vi "Initialize.vi"(8 "error in (no error)":errorcluster, 9 "Reset (True)":bool=TRUE, 10 "ID Query (True)":bool=TRUE, 11 "VISA resource name":refnum<visa-resource-name>) -> (0 "error out":errorcluster, 3 "VISA resource name out":refnum<visa-resource-name>)   [LabVIEW 2020, in "Library Instrument & Equipement.lvlib" / "Library Multimeter.lvlib" / "RIGOL DM3058.lvlib"]
doc: "Establishes communication with the instrument and optionally performs an instrument identification query and/or an instrument reset. It also places the instrument in a default state needed for other instrument driver operations. Therefore, call this VI before calling other instrument driver VIs for this instrument. Generally, you need to call the Initialize VI only once at the beginning of an application."
uses:
  RIGOL DM3058.lvlib
panel:
  # "(c) 2009-2015, RIGOL Technologies, Inc.  All Rights Reserved."
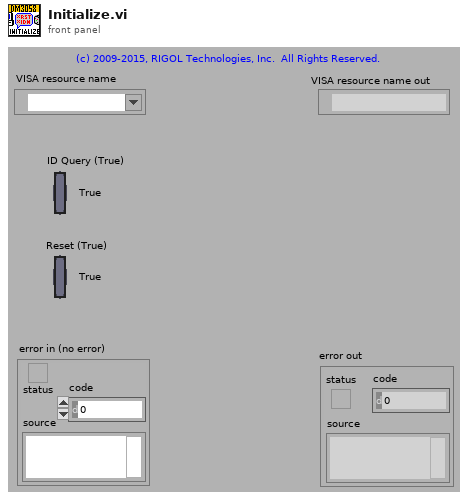
[diagram p1: front panel]
types:
  T1 = cluster{"DM Series Mode":u16, "Measurement Function":u16}
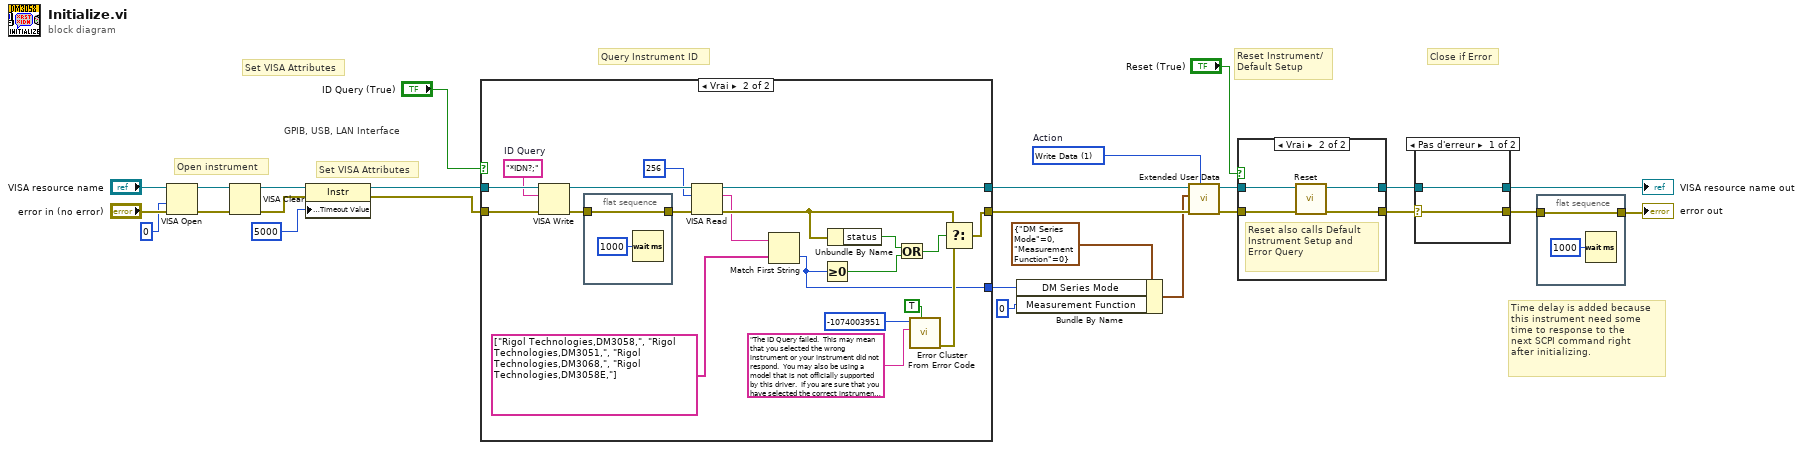
[diagram p0: block diagram]
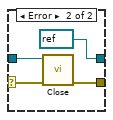
[diagram p2: hidden frame]
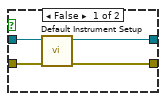
[diagram p3: hidden frame]
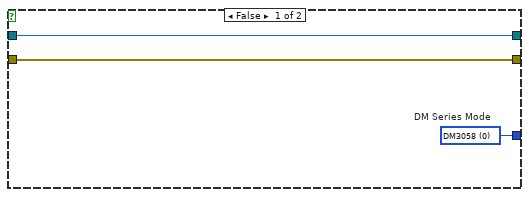
[diagram p4: hidden frame]
diagram:
  w9 = 1 items=["Read Data", "Write Data", "Clear Data", "Clear ALL Data"]  # Action
  # "Time delay is added because \nthis instrument need some \ntime to response to the \nnext SCPI command right \nafter initializing."
  # "Set VISA Attributes"
  # "GPIB, USB, LAN Interface"
  # "Set VISA Attributes"
  # "Close if Error"
  # "Query Instrument ID"
  # "Reset Instrument/\nDefault Setup"
  # "Open instrument"
  n1 = VISA Open(access mode=u32 0, error in (no error)="error in (no error)", VISA resource name="VISA resource name") -> (VISA resource name=w20:refnum<visa-resource-name>, error out=w19:errorcluster)  [unwired: 2 out]
  n2 = VISA Clear(VISA resource name=w20, error in (no error)=w19) -> (VISA resource name out=w18:refnum<visa-resource-name>, error out=w17:errorcluster)
  n3 = property class="Instr"(reference=w18, error in=w17, "General Settings:Timeout Value"=u32 5000) -> (reference out=w5:refnum<visa-resource-name>, error out=w4:errorcluster)
  n4 = case shown="Vrai" "ID Query (True)" {
    tunnel: [w28 w49] -> w12
    tunnel: [w29 w46] -> w13
    tunnel: w5 -> [w29 w47]
    tunnel: w4 -> [w28 w48]
    tunnel: [w27 w32] -> w8
    frame False {
      w27 = u16 0 items=["DM3058", "DM3051", "DM3068"]  # DM Series Mode
    }
    frame True {
      w43 = "*IDN?;"  # ID Query
      n5 = VISA Write(VISA resource name=w47, write buffer=w43, error in (no error)=w48) -> (VISA resource name out=w45:refnum<visa-resource-name>, error out=w30:errorcluster)  [unwired: 1 out]
      n6 = flat-sequence {
        tunnel: w30 -> [w51]
        tunnel: [w51] -> w31
        frame #0 {
          n7 = Wait (ms)(milliseconds to wait=u32 1000) -> ()  [unwired: 1 out]
        }
      }
      n8 = VISA Read(VISA resource name=w45, byte count=u32 256, error in (no error)=w31) -> (VISA resource name out=w46:refnum<visa-resource-name>, read buffer=w33:string, error out=w38:errorcluster)  [unwired: 1 out]
      n9 = Match First String(2:string[] ["Rigol Technologies,DM3058,", "Rigol Technologies,DM3051,", "Rigol Technologies,DM3068,", "Rigol Technologies,DM3058E,"], 3:w33) -> (0:w32:i32)  [unwired: 1 out]
      n10 = Greater Or Equal To 0?(x=w32) -> (x >= 0?=w36:bool)
      n11 = Unbundle By Name(w38) -> ("status"=w37:bool)
      n12 = Or(x=w37, y=w36) -> (x .or. y?=w35:bool)
      n13 = call <vilib>:"Error Cluster From Error Code.vi"("show call chain? (False)"=TRUE, "error message (\"\")"="The ID Query failed.  This may mean that you selected the wrong instrument or your instrument did not respond.  You may also be using a model that is not officially supported by this driver.  If you are sure that you have selected the correct instrument and it is responding, try disabling the ID Query." ("Source (VI Name)"), "error code (0)"=-1074003951 ("Code")) -> ("error out"=w42:errorcluster)  [unwired: 1 in, 5 out]
      n14 = Select(t=w38, s=w35, f=w42) -> (s? t:f=w49:errorcluster)
    }
  }
  n15 = Bundle By Name(cluster=T1 {"DM Series Mode"=0, "Measurement Function"=0} ("User Data In"), "DM Series Mode"=w8, "Measurement Function"=u16 0) -> (w7:T1)
  n16 = call "Extended User Data.vi"("Action (1: Write Data)"=w9, "Error In (no error)"=w12, "User Data In"=w7, "VISA resource name in"=w13) -> ("Error Out"=w11:errorcluster, "VISA resource name out"=w10:refnum<visa-resource-name>)  [unwired: 6 out]
  n17 = case shown="Vrai" "Reset (True)" {
    tunnel: w11 -> [w54 w56]
    tunnel: [w52 w59] -> w14
    tunnel: w10 -> [w55 w57]
    tunnel: [w53 w58] -> w15
    frame False {
      n18 = call "Default Instrument Setup.vi"("error in (no error)"=w54, "VISA resource name"=w55) -> ("error out"=w52:errorcluster, "VISA resource name out"=w53:refnum<visa-resource-name>)  [unwired: 8 out]
    }
    frame True {
      # "Reset also calls Default Instrument Setup and Error Query"
      n19 = call "Reset.vi"("error in (no error)"=w56, "VISA resource name"=w57) -> ("error out"=w59:errorcluster, "VISA resource name out"=w58:refnum<visa-resource-name>)  [unwired: 8 out]
    }
  }
  n20 = case shown="Pas d'erreur" w14 {
    selector: w14 -> [w60 w63]
    tunnel: w15 -> [w61 w64]
    tunnel: [w61 refnum<visa-resource-name> refnum ("VISA resource name out")] -> w16
    tunnel: [w60 w65] -> w2
    frame No Error {
    }
    frame Error {
      n21 = call "Close.vi"("error in (no error)"=w63, "VISA resource name"=w64) -> ("error out"=w65:errorcluster)  [unwired: 9 out]
    }
  }
  "VISA resource name out" <- w16
  n22 = flat-sequence {
    tunnel: w2 -> [w67]
    tunnel: [w67] -> w3
    frame #0 {
      n23 = Wait (ms)(milliseconds to wait=u32 1000) -> ()  [unwired: 1 out]
    }
  }
  "error out" <- w3
